vi "_Clear MulticolumnListbox - FP.vi"(0 "GObject in":refnum<vi>, 5 "error in (no error)":errorcluster) -> (14 "changed?":bool, 19 "error out":errorcluster)   [LabVIEW 2015, in "QD_Erease Data.lvlib"]
uses:
  QD_Erease Data.lvlib
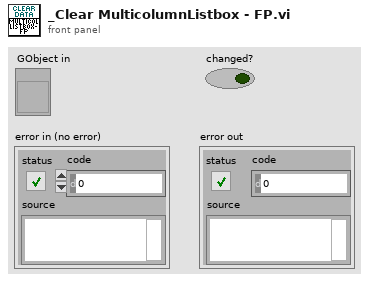
[diagram p1: front panel]
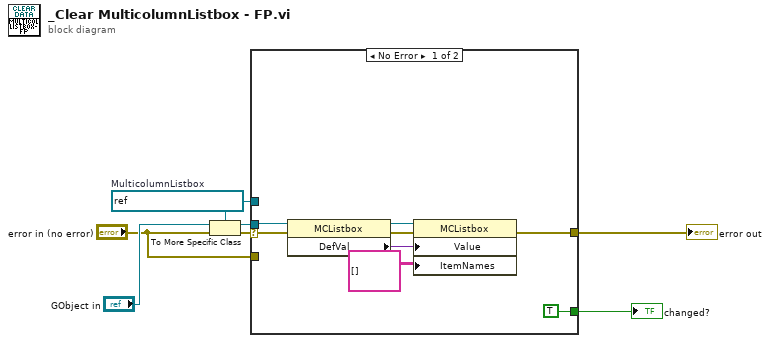
[diagram p0: block diagram]
diagram:
  w1 = refnum<vi> refnum  # MulticolumnListbox
  n1 = To More Specific Class(target class=w1, reference="GObject in", error in="error in (no error)") -> (specific class reference=w3:refnum<vi>, error out=w4:errorcluster)
  n2 = case shown="No Error" w4 {
    selector: w4 -> [w8 _]
    tunnel: [w15 w16] -> w2
    tunnel: w3 -> [w9 _]
    tunnel: "error in (no error)" -> [_ w16]
    tunnel: [TRUE _] -> w7
    tunnel: w1 -> [_ _]
    frame No Error {
      n3 = property class="MCListbox"(reference=w9, error in=w8) -> (reference out=w13:refnum<vi>, error out=w12:errorcluster, "DefVal"=w11:variant)
      n4 = property class="MCListbox"(reference=w13, error in=w12, "Value"=w11, "ItemNames"=string[][] [] ("Item Names")) -> (error out=w15:errorcluster)  [unwired: 1 out]
    }
    frame Error {
    }
  }
  "changed?" <- w7
  "error out" <- w2
